vi "FormatResponse.vi"(10 "JSON Error Strings":string[](array[string]), 11 "JSON Response Strings":string[](array[string])) -> (1 "ResponseWithLength":string, 2 "ResponseLength":i32, 3 "FormattedResponse":string)   [LabVIEW 2013]
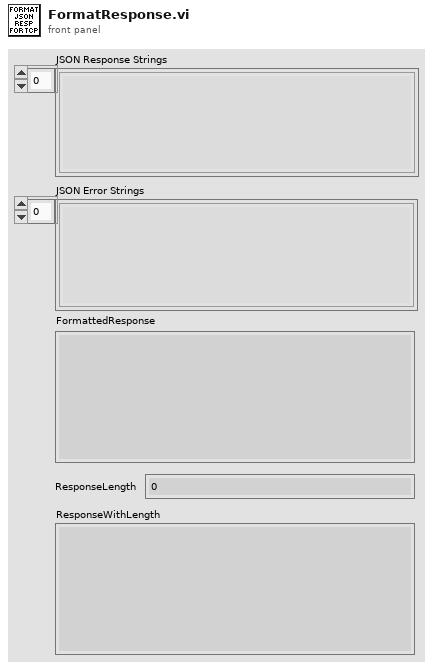
[diagram p1: front panel]
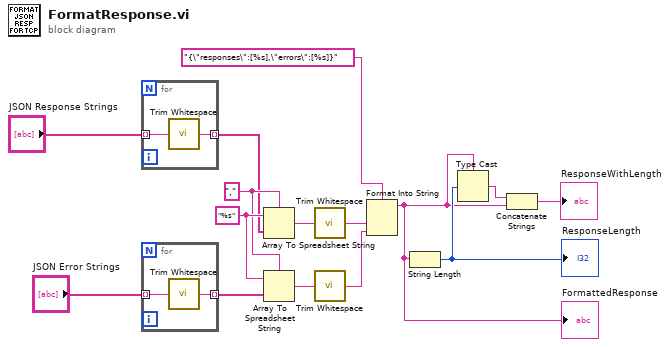
[diagram p0: block diagram]
diagram:
  w12 = "," ("delimiter (Tab)")
  w13 = "%s" ("format string")
  n1 = for {
    tunnel: "JSON Response Strings" -> [w17] mode=indexing
    tunnel: [w16] -> w10 mode=indexing
    n2 = call <vilib>:"Trim Whitespace.vi"("string"=w17) -> ("trimmed string"=w16:string)  [unwired: 1 in]
  }
  n3 = for {
    tunnel: "JSON Error Strings" -> [w19] mode=indexing
    tunnel: [w18] -> w11 mode=indexing
    n4 = call <vilib>:"Trim Whitespace.vi"("string"=w19) -> ("trimmed string"=w18:string)  [unwired: 1 in]
  }
  n5 = Array To Spreadsheet String(delimiter (Tab)=w12, array=w10, 3:w13) -> (spreadsheet string=w9:string)
  n6 = Array To Spreadsheet String(delimiter (Tab)=w12, array=w11, 3:w13) -> (spreadsheet string=w8:string)
  n7 = call <vilib>:"Trim Whitespace.vi"("string"=w9) -> ("trimmed string"=w6:string)  [unwired: 1 in]
  n8 = call <vilib>:"Trim Whitespace.vi"("string"=w8) -> ("trimmed string"=w5:string)  [unwired: 1 in]
  n9 = Format Into String(format string="{\"responses\":[%s],\"errors\":[%s]}", w6, w5) -> (resulting string=w2:string)  [unwired: 2 in, 1 out]
  "FormattedResponse" <- w2
  n10 = String Length(string=w2) -> (length=w4:i32)
  "ResponseLength" <- w4
  n11 = Type Cast(type=w2, x=w4) -> (*(type *) &x=w3:string)
  n12 = Concatenate Strings(w3, w2) -> (→"ResponseWithLength":string)
